vi "QCA - DUT Generate Rx Configuration.vi"(0 "Mac Address":string, 11 "error in (no error)":errorcluster, 13 "Rx_Test Parameters":T3 {"OFDM Data Rate (Mbps)" items=["6", "9", "12", "18", "24", "36", "48", "54"]; "DSSS Data Rate (Mbps)" items=["1", "2", "5.5 CCK", "5.5 PBCC", "11 CCK", "11 PBCC", "22", "33"]; "80211n PLCP Frame Format" items=["Mixed Format", "Greenfield Format"]}) -> (4 "RateSet_r":i32[](array[numeric]), 8 "Rx Configuration":T2, 15 "error out":errorcluster)   [LabVIEW 2011]
uses:
  TV/RW/Includes/WLAN - TV - RW - INC - RxTestParameters.ctl
  Controls/Data Rates.ctl
panel:
  in  "OFDM Data Rate (Mbps)":i32(ring) items=["6", "9", "12", "18", "24", "36", "48", "54"]
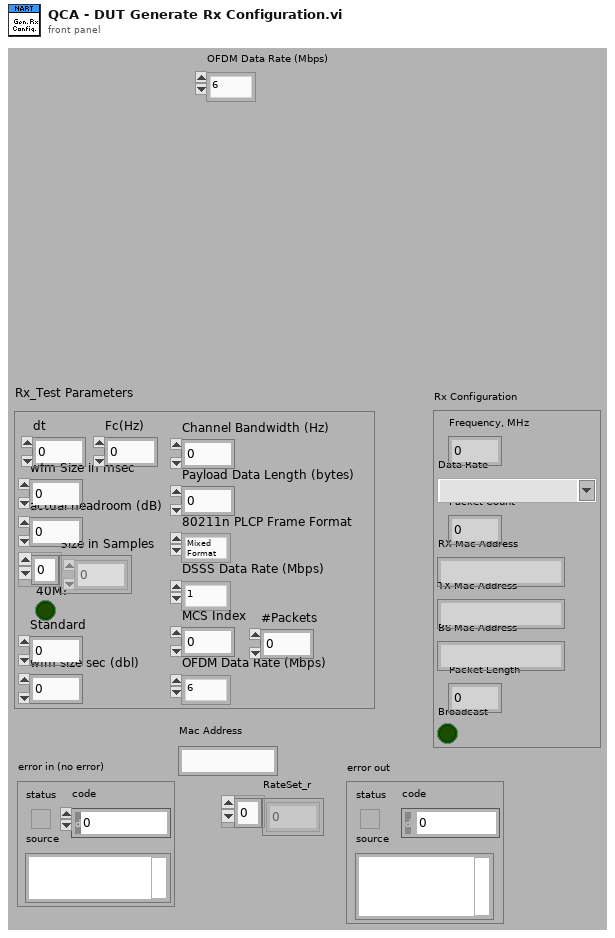
[diagram p1: front panel]
types:
  T1 = typedef "Data Rates.ctl" = string
  T2 = cluster{"Frequency, MHz":u32, "Data Rate":T1, "Packet Count":i32, "RX Mac Address":string, "TX Mac Address":string, "BS Mac Address":string, "Packet Length":u32, "Broadcast":bool}
  T3 = typedef "WLAN - TV - RW - INC - RxTestParameters.ctl" = cluster{"wfm Size in msec":i32, "actual headroom (dB)":dbl, "Size in Samples":i32[], "40M?":bool, "Standard ":i32, "wfm size sec (dbl)":dbl, "dt":dbl, "Channel Bandwidth (Hz)":dbl, "Payload Data Length (bytes)":i32, "80211n PLCP Frame Format":i32, "DSSS Data Rate (Mbps)":i32, "OFDM Data Rate (Mbps)":i32, "MCS Index":i32, "Fc(Hz)":dbl, "#Packets":i32}
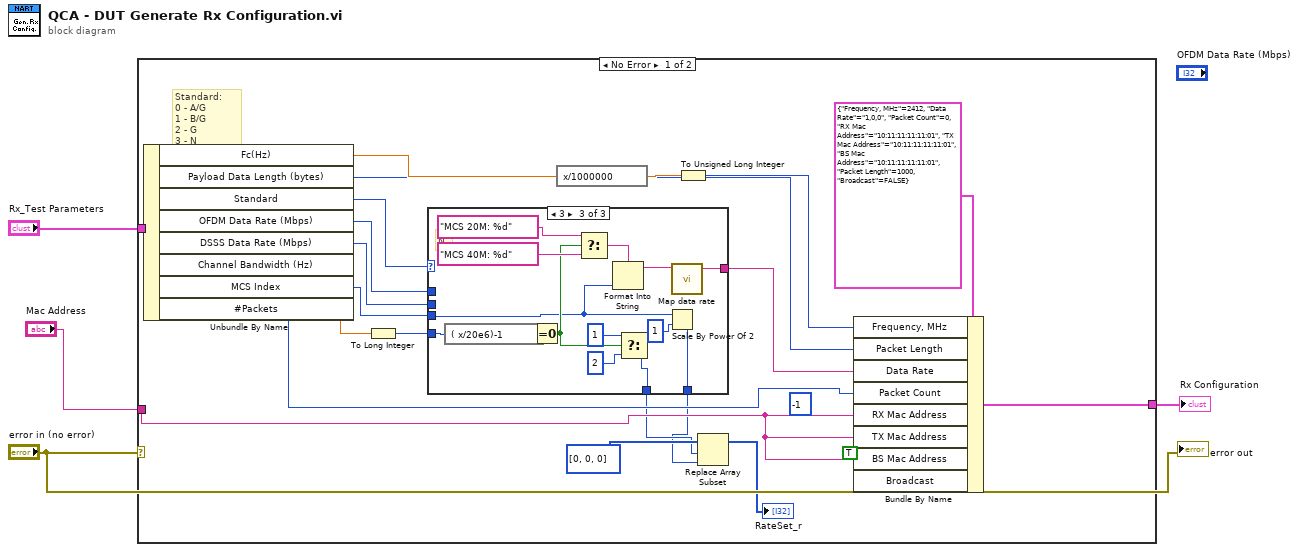
[diagram p0: block diagram]
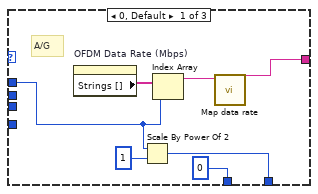
[diagram p2: hidden frame]
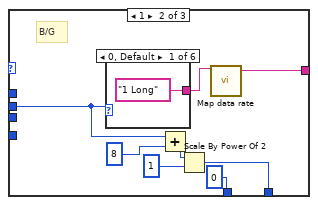
[diagram p3: hidden frame]
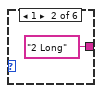
[diagram p4: hidden frame]
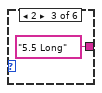
[diagram p5: hidden frame]
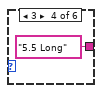
[diagram p6: hidden frame]
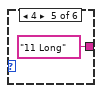
[diagram p7: hidden frame]
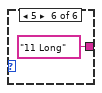
[diagram p8: hidden frame]
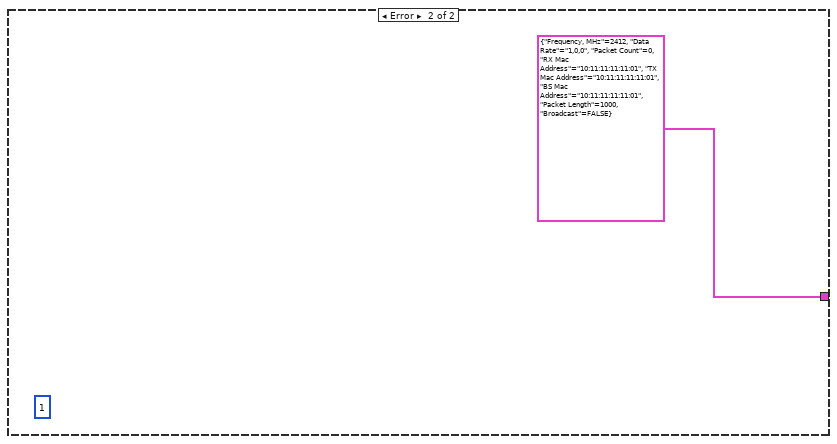
[diagram p9: hidden frame]
diagram:
  n1 = case shown="No Error" "error in (no error)" {
    tunnel: "Rx_Test Parameters" -> [w22 _]
    tunnel: [w15 T2 {"Frequency, MHz"=2412, "Data Rate"="1,0,0", "Packet Count"=0, "RX Mac Address"="10:11:11:11:11:01", "TX Mac Address"="10:11:11:11:11:01", "BS Mac Address"="10:11:11:11:11:01", "Packet Length"=1000, "Broadcast"=FALSE} ("Receive Config")] -> w3
    tunnel: "Mac Address" -> [w9 _]
    frame No Error {
      (unwired) -1 ("Packet Count")
      # "Standard:\n0 - A/G\n1 - B/G\n2 - G\n3 - N"
      n2 = Unbundle By Name(w22) -> ("Fc(Hz)"=w13:dbl, "Payload Data Length (bytes)"=w12:i32, "Standard"=w21:i32, "OFDM Data Rate (Mbps)"=w20:i32, "DSSS Data Rate (Mbps)"=w19:i32, "Channel Bandwidth (Hz)"=w14:dbl, "MCS Index"=w18:i32, "#Packets"=w10:i32)
      n3 = To Long Integer(number=w14) -> (32bit integer=w11:i32)
      n4 = case shown="3" w21 {
        tunnel: w20 -> [w26 _ _]
        tunnel: w19 -> [_ w33 _]
        tunnel: w18 -> [_ _ w50]
        tunnel: [w32 w40 w60] -> w17
        tunnel: w11 -> [_ _ w58]
        tunnel: [0 0 w48] -> w7
        tunnel: [w27 w34 w47] -> w6
        frame 0, Default {
          # "A/G"
          n5 = property on="OFDM Data Rate (Mbps)" class="Ring (strict)"() -> ("Strings []"=w31:string[])  [unwired: 2 in, 2 out]
          n6 = Scale By Power Of 2(n=w26, x=1) -> (x*2^n=w27:i32)
          n7 = Index Array(array=w31, index=w26) -> (element=w30:string)
          n8 = call "Map data rate.vi"("Data Rate In"=w30) -> ("Data Rate Out"=w32:string)  [unwired: 10 in]
        }
        frame 1 {
          # "B/G"
          n9 = case shown="0, Default" w33 {
            tunnel: ["1 Long" ("Data Rate In") "2 Long" ("Data Rate In") "5.5 Long" ("Data Rate In") "5.5 Long" ("Data Rate In") "11 Long" ("Data Rate In") "11 Long" ("Data Rate In")] -> w39
            frame 0, Default {
            }
            frame 1 {
            }
            frame 2 {
            }
            frame 3 {
            }
            frame 4 {
            }
            frame 5 {
            }
          }
          n10 = Add(x=w33, y=8) -> (x+y=w38:i32)
          n11 = Scale By Power Of 2(n=w38, x=1) -> (x*2^n=w34:i32)
          n12 = call "Map data rate.vi"("Data Rate In"=w39) -> ("Data Rate Out"=w40:string)  [unwired: 10 in]
        }
        frame 3 {
          # "N"
          n13 = expression code="( x/20e6)-1"(w58) -> (w55:i32)
          n14 = Equal To 0?(x=w55) -> (x = 0?=w51:bool)
          n15 = Select(t="MCS 20M: %d" ("format string"), s=w51, f="MCS 40M: %d" ("format string")) -> (s? t:f=w54:string)
          n16 = Format Into String(format string=w54, w50) -> (resulting string=w59:string)  [unwired: 2 in, 1 out]
          n17 = Select(t=1, s=w51, f=2) -> (s? t:f=w48:i32)
          n18 = Scale By Power Of 2(n=w50, x=1) -> (x*2^n=w47:i32)
          n19 = call "Map data rate.vi"("Data Rate In"=w59) -> ("Data Rate Out"=w60:string)  [unwired: 10 in]
        }
      }
      n20 = expression code="x/1000000"(w13) -> (w24:dbl)
      n21 = To Unsigned Long Integer(number=w24) -> (unsigned 32bit integer=w23:u32)
      n22 = Replace Array Subset(array=i32[] [0, 0, 0], new element=w6, index=w7) -> (→"RateSet_r":i32[])
      n23 = Bundle By Name(cluster=T2 {"Frequency, MHz"=2412, "Data Rate"="1,0,0", "Packet Count"=0, "RX Mac Address"="10:11:11:11:11:01", "TX Mac Address"="10:11:11:11:11:01", "BS Mac Address"="10:11:11:11:11:01", "Packet Length"=1000, "Broadcast"=FALSE} ("Receive Config"), "Frequency, MHz"=w23, "Packet Length"=w12, "Data Rate"=w17, "Packet Count"=w10, "RX Mac Address"=w9, "TX Mac Address"=w9, "BS Mac Address"=w9, "Broadcast"=TRUE ("ART2 Data.Receive Config.Broadcast")) -> (w15:T2)
    }
    frame Error {
      (unwired) 1 ("Rx_Chan")
    }
  }
  "Rx Configuration" <- w3
  "error out" <- "error in (no error)"
